vi "Cancel Subscribe.vi"(8 "error in (no error)":errorcluster, 10 "Subscriber In":refnum<class "Subscriber.lvclass">, 11 "Observer in":refnum<class "Observer.lvclass">) -> (0 "error out":errorcluster, 3 "Observer out":refnum<class "Observer.lvclass">)   [LabVIEW 2019, in "Observer.lvclass"]
uses:
  Observer.lvclass
  Subscriber/Subscriber.lvclass
  Observer.lvclass/Observer.ctl
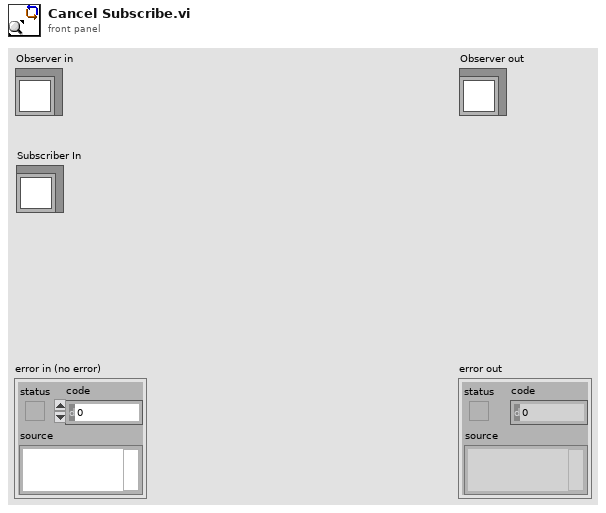
[diagram p1: front panel]
types:
  T1 = typedef "Subcribe Set.ctl" = set{refnum<class "Subscriber.lvclass">}
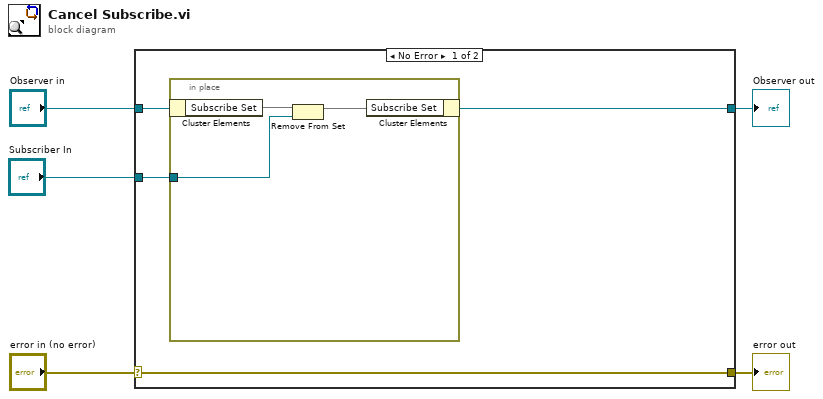
[diagram p0: block diagram]
diagram:
  n1 = case shown="No Error" "error in (no error)" {
    selector: "error in (no error)" -> [w9 w14]
    tunnel: [w9 w14] -> w4
    tunnel: [w7 w13] -> w2
    tunnel: "Observer in" -> [w8 w13]
    tunnel: "Subscriber In" -> [w6 _]
    frame No Error {
      n2 = in-place {
        in-place-border: w6 -> [w10]
        n3 = in-place-cluster #1(w8) -> ("Subscribe Set"=w12:T1)
        n4 = Remove From Set(10:w10, 11:w12) -> (3:w11:T1)  [unwired: 1 out]
        n5 = in-place-cluster #1("Subscribe Set"=w11) -> (w7:refnum<class "Observer.lvclass">)
      }
    }
    frame Error {
    }
  }
  "error out" <- w4
  "Observer out" <- w2
